vi "Intake.vi"(8 "error in (no error)":errorcluster, 9 "Out":bool, 10 "In":bool, 11 "Cargo in":refnum<class "Cargo Concrete.lvclass">) -> (0 "error out":errorcluster, 3 "Cargo out":refnum<class "Cargo Concrete.lvclass">)   [LabVIEW 2019, in "Cargo.lvlib" / "Cargo Concrete.lvclass"]
doc: "This VI sets the motor outputs intake based on state."
uses:
  Cargo Concrete.lvclass
  C:/Users/rishi/OneDrive/Documents/2020InfinteRecharge/src robot/Classes/Cargo/Cargo.lvclass
  Cargo Concrete.lvclass/Cargo Concrete.ctl
  Cargo.lvclass
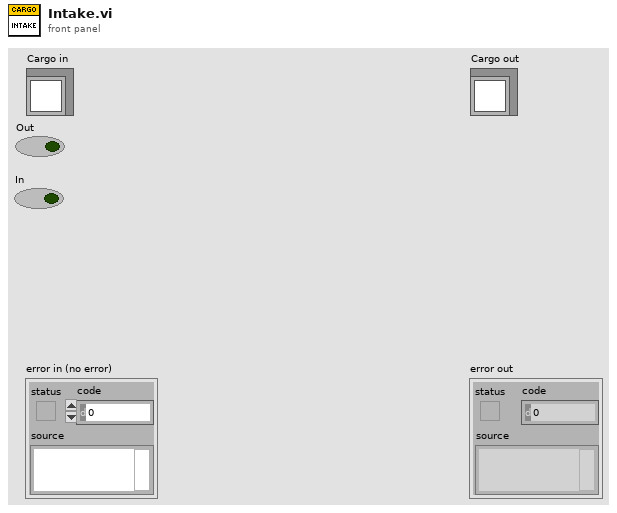
[diagram p1: front panel]
types:
  T1 = typedef "Cargo.lvlib/Cargo.lvclass/Cargo States.ctl" = enum16{"Off", "Intake Full", "Intake Idle", "Output Full"}
  T2 = typedef "WPI_MotorControlDeviceRef.ctl" = cluster{"DeviceStatus":errorcluster, "Type":T3, "PWM":cluster{"PWM Channel":T4, "DeadBand":T5}, "CAN":cluster{"Device Number":u8, "SetOutput VI Ref":variant, "GetOutput VI Ref":variant, "Enable VI Ref":variant, "Disable VI Ref":variant, "Data":variant}, "Invert":bool, "DIO PWM":cluster{"PWM \"Enable\" Channel":T4, "DIOChannel":T6, "PWM Rate":dbl}}
  T3 = typedef "WPI_MotorControlType.ctl" = enum16{"PWM", "CAN", "DIO PWM"}
  T4 = typedef "FPGA_DIOPWMChannel.ctl" = enum8{"PWM 0", "PWM 1", "PWM 2", "PWM 3", "PWM 4", "PWM 5", "PWM 6", "PWM 7", "PWM 8", "PWM 9", "PWM MXP 0", "PWM MXP 1", "PWM MXP 2", "PWM MXP 3", "PWM MXP 4", "PWM MXP 5", "PWM MXP 6", "PWM MXP 7", "PWM MXP 8", "PWM MXP 9", "Invalid"}
  T5 = typedef "WPI_PWMDeadband.ctl" = cluster{"Name":string, "maxPositivePwm":i32, "minPositivePwm":i32, "centerPwm":i32, "maxNegativePwm":i32, "minNegativePwm":i32, "angularRange":u16}
  T6 = typedef "FPGA_DIOChannel.ctl" = enum8{"DIO 0", "DIO 1", "DIO 2", "DIO 3", "DIO 4", "DIO 5", "DIO 6", "DIO 7", "DIO 8", "DIO 9", "DIO MXP 0", "DIO MXP 1", "DIO MXP 2", "DIO MXP 3", "DIO MXP 4", "DIO MXP 5", "DIO MXP 6", "DIO MXP 7", "DIO MXP 8", "DIO MXP 9", "DIO MXP 10", "DIO MXP 11", "DIO MXP 12", "DIO MXP 13", "DIO MXP 14", "DIO MXP 15", "SPI Port CS1", "SPI Port CS2", "SPI Port CS3", "SPI Port MISO", "SPI Port MOSI", "Invalid"}
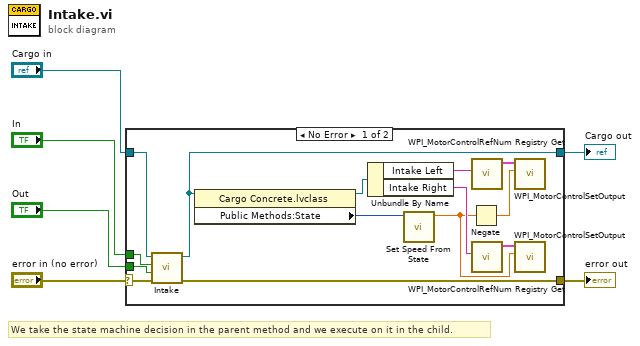
[diagram p0: block diagram]
diagram:
  # "We take the state machine decision in the parent method and we execute on it in the child."
  n1 = case shown="No Error" "error in (no error)" {
    selector: "error in (no error)" -> [w19 w22]
    tunnel: [w20 w22] -> w6
    tunnel: [w11 w21] -> w5
    tunnel: "Cargo in" -> [w13 w21]
    tunnel: "In" -> [w10 _]
    tunnel: "Out" -> [w9 _]
    frame No Error {
      n2 = call-parent "Intake.vi"("error in (no error)"=w19, "Out"=w9, "In"=w10, "Cargo in"=w13) -> ("error out"=w20:errorcluster, "Cargo out"=w11:refnum<class "Cargo Concrete.lvclass">)  [unwired: 6 in]
      n3 = property class="Cargo Concrete.lvclass"(reference=w11) -> (reference out=w12:refnum<class "Cargo Concrete.lvclass">, "Public Methods:State"=w14:T1)  [unwired: 1 in, 1 out]
      n4 = Unbundle By Name(w12) -> ("Intake Left"=w18:string, "Intake Right"=w17:string)
      n5 = call "Set Speed From State.vi"("Public Methods:State"=w14) -> ("Output"=w7:dbl)  [unwired: 10 in]
      n6 = Negate(x=w7) -> (-x=w8:dbl)
      n7 = call <vilib>:"WPI_MotorControlRefNum Registry Get.vi"("refnum name"=w18) -> ("MotorControlDevRef"=w16:T2)  [unwired: 9 in, 1 out]
      n8 = call <vilib>:"WPI_MotorControlRefNum Registry Get.vi"("refnum name"=w17) -> ("MotorControlDevRef"=w15:T2)  [unwired: 9 in, 1 out]
      n9 = call <vilib>:"WPI_MotorControlSetOutput.vi"("Output"=w8, "MotorControlDevRef"=w16) -> ()  [unwired: 7 in, 3 out]
      n10 = call <vilib>:"WPI_MotorControlSetOutput.vi"("Output"=w7, "MotorControlDevRef"=w15) -> ()  [unwired: 7 in, 3 out]
    }
    frame Error {
    }
  }
  "error out" <- w6
  "Cargo out" <- w5
